vi "allValsCtor.vi"(8 "error in (no error)":errorcluster, 9 "Default Data Value":variant, 10 "Allowed Robot Modes":string[](array[string]), 11 "Name":string) -> (0 "error out":errorcluster, 3 "Command out":refnum<class "Command.lvclass">)   [LabVIEW 2017, in "Command.lvclass"]
uses:
  <userlib>/836-Library/Robot/Command/Command.lvclass
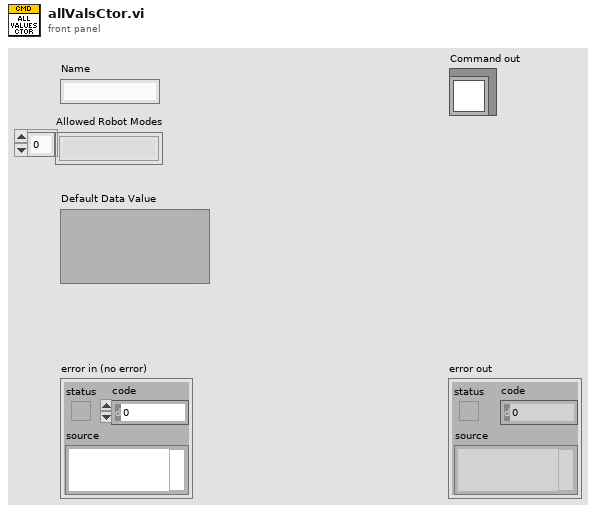
[diagram p1: front panel]
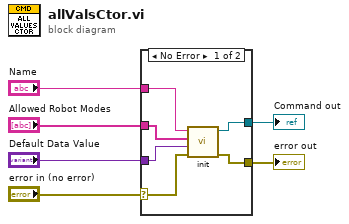
[diagram p0: block diagram]
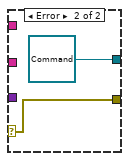
[diagram p2: hidden frame]
diagram:
  n1 = case shown="No Error" "error in (no error)" {
    selector: "error in (no error)" -> [w9 w14]
    tunnel: [w8 w14] -> w5
    tunnel: "Name" -> [w12 _]
    tunnel: "Allowed Robot Modes" -> [w11 _]
    tunnel: "Default Data Value" -> [w10 _]
    tunnel: [w7 refnum<class "Command.lvclass"> refnum ("Command out")] -> w1
    frame No Error {
      n2 = call <userlib>:"init.vi"("error in (no error)"=w9, "Default Data"=w10, "Allowed Robot Modes"=w11, "Name"=w12) -> ("error out"=w8:errorcluster, "Command out"=w7:refnum<class "Command.lvclass">)  [unwired: 6 in]
    }
    frame Error {
    }
  }
  "error out" <- w5
  "Command out" <- w1
